vi "格式时间字符串.vi"(11 "字符串":string) -> (3 "连接的字符串":string)   [LabVIEW 2016]
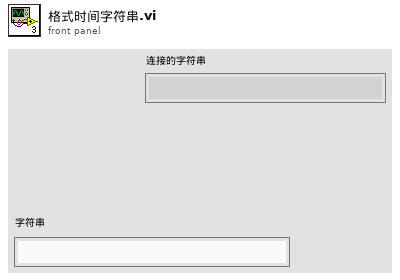
[diagram p1: front panel]
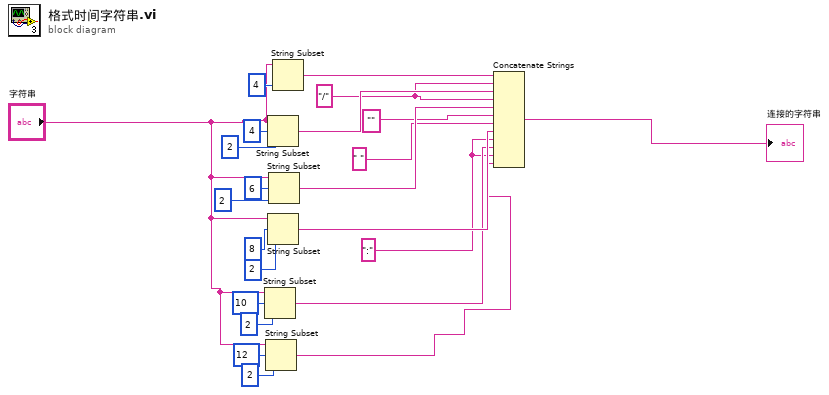
[diagram p0: block diagram]
diagram:
  w8 = ":" ("子字符串;substring")
  w13 = "/" ("子字符串;substring")
  n1 = String Subset(string="字符串", offset (0)=10 ("偏移量(0)"), length (rest)=2 ("长度（剩余）")) -> (substring=w9:string)
  n2 = String Subset(string="字符串", offset (0)=12 ("偏移量(0)"), length (rest)=2 ("长度（剩余）")) -> (substring=w4:string)
  n3 = String Subset(string="字符串", offset (0)=4 ("偏移量(0)"), length (rest)=2 ("长度（剩余）")) -> (substring=w15:string)
  n4 = String Subset(string="字符串", offset (0)=8 ("偏移量(0)"), length (rest)=2 ("长度（剩余）")) -> (substring=w12:string)
  n5 = String Subset(string="字符串", offset (0)=6 ("偏移量(0)"), length (rest)=2 ("长度（剩余）")) -> (substring=w14:string)
  n6 = String Subset(string="字符串", length (rest)=4 ("长度（剩余）")) -> (substring=w16:string)  [unwired: 1 in]
  n7 = Concatenate Strings(w16, w13, w15, w13, w14, "", " " ("子字符串;substring"), w12, w8, w9, w8, w4) -> (→"连接的字符串":string)
